vi "Wire Inputs.vi"(8 "error in (no error)":errorcluster, 9 "Inputs":refnum<vi>[](array[refnum]), 10 "Names":string[](array[string]), 11 "Node in":refnum<vi>) -> (0 "error out":errorcluster, 3 "Node out":refnum<vi>)   [LabVIEW 2015, in "Scripting.lvlib"]
uses:
  Scripting.lvlib
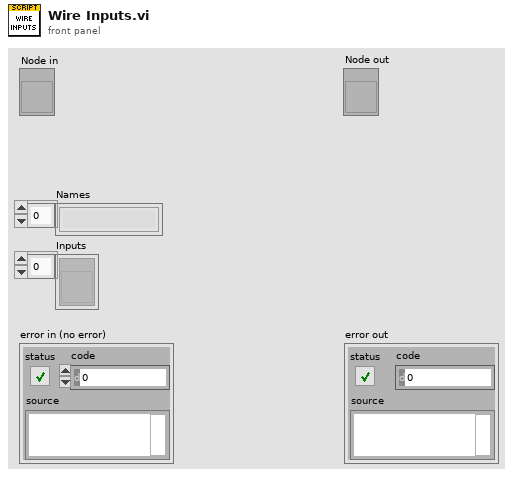
[diagram p1: front panel]
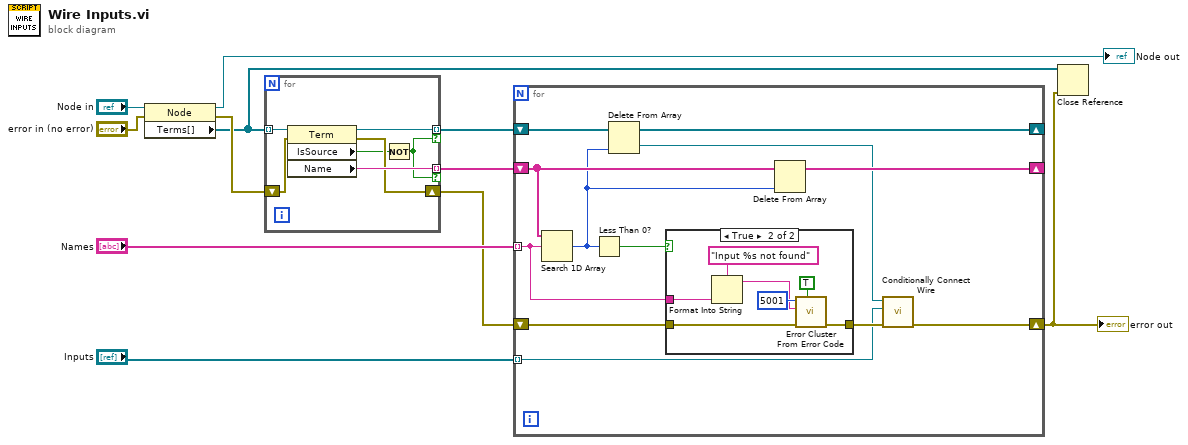
[diagram p0: block diagram]
diagram:
  n1 = property class="Node"(reference="Node in", error in="error in (no error)") -> (reference out=→"Node out":refnum<vi>, error out=w6:errorcluster, "Terms[]"=w2:refnum<vi>[])
  n2 = for {
    tunnel: w2 -> [w18] mode=indexing
    tunnel: [w13] -> w9 mode=indexing if=w16
    tunnel: [w17] -> w8 mode=indexing if=w16
    shift-right: [w14] -> w3
    shift-left: w6 -> [w15]
    n3 = property class="Term"(reference=w18, error in=w15) -> (reference out=w13:refnum<vi>, error out=w14:errorcluster, "IsSource"=w12:bool, "Name"=w17:string)
    n4 = Not(x=w12) -> (.not. x?=w16:bool)
  }
  n5 = for {
    tunnel: "Names" -> [w27] mode=indexing
    shift-right: [w19] -> w1
    shift-left: w3 -> [w28]
    shift-right: [w24] -> _
    shift-left: w8 -> [w26]
    tunnel: "Inputs" -> [w20] mode=indexing
    shift-right: [w23] -> _
    shift-left: w9 -> [w30]
    n6 = Search 1D Array(1D array=w26, element=w27) -> (index of element=w25:i32)  [unwired: 1 in]
    n7 = Less Than 0?(x=w25) -> (x < 0?=w29:bool)
    n8 = Delete From Array(array=w30, index=w25) -> (deleted portion=w21:refnum<vi>, array with subset deleted=w23:refnum<vi>[])  [unwired: 1 in]
    n9 = case shown="True" w29 {
      tunnel: w28 -> [w31 w37]
      tunnel: w27 -> [_ w35]
      tunnel: [w31 w32] -> w22
      frame False {
      }
      frame True {
        n10 = Format Into String(format string="Input %s not found", w35) -> (resulting string=w34:string)  [unwired: 2 in, 1 out]
        n11 = call <vilib>:"Error Cluster From Error Code.vi"("show call chain? (False)"=TRUE, "error in (no error)"=w37, "error message (\"\")"=w34, "error code (0)"=5001) -> ("error out"=w32:errorcluster)  [unwired: 5 in]
      }
    }
    n12 = Delete From Array(array=w26, index=w25) -> (array with subset deleted=w24:string[])  [unwired: 1 in, 1 out]
    n13 = call "Conditionally Connect Wire.vi"("error in (no error)"=w22, "Wire Source"=w20, "Terminal in"=w21) -> ("error out"=w19:errorcluster)  [unwired: 7 in, 1 out]
  }
  "error out" <- w1
  n14 = Close Reference(reference=w2, error in (no error)=w1) -> ()  [unwired: 1 out]
